vi "ep_Private Inf to Task.vi"(5 "entry values":string[](array[string]), 7 "entry names":string[](array[string]), 8 "error in":errorcluster, 9 "section name":string, 10 "manufacturer name":string, 11 "task in":T1={"file refnums"=[], "Data Object"=refnum, "config info"={"station_name"="", "rec_dev_id"="", "rev_year"=1999.0, "TT"=0, "##A"=0, "##D"=0, "analog channel info"=[], "status channel info"=[], "lf"=-inf, "nrates"=65535, "samp info"=[], "initial timestamp"=timestamp(0 s since 1904-01-01), "trigger timestamp"=timestamp(0 s since 1904-01-01), "ft"=enum."Binary", "timemult"=1.0}, "public inf content"={"Source"="", "Record Type"=enum."Fault", "Phase ID"="", "Event Description"="", "Device ID"="", "Distance of Fault"=-1.0, "Distance Unit"=enum."Miles", "Max_Current"=inf, "Min_Current"=-inf, "Max_Voltage"=inf, "Min_Voltage"=-inf, "EventNoteCount"=0, "Event Information"=[]}, "private inf content"=[], "internal buffers"={"start index"=1, "config to public inf"=enum."disabled", "static config info"="", "static file_des record inf"="", "static file_des channel inf"="", "public inf"="", "private inf"=""}} {"public inf content"."Event Information"."min sample number" max=9999999999; "public inf content"."Event Information"."max sample number" max=9999999999; "config info"."nrates" max=999; "config info"."status channel info"."Dn" min=1 max=999999; "config info"."analog channel info"."An" min=1 max=999999; "config info"."trigger timestamp" format="%<%H:%M:%S%6u\n%d/%m/%Y>T"; "config info"."initial timestamp" format="%<%H:%M:%S%6u\n%d/%m/%Y>T"; "config info"."##D" max=999999; "config info"."##A" max=999999; "config info"."TT" min=1 max=999999; "config info"."rev_year" min=1999.0 max=1999.0}) -> (0 "error out":errorcluster, 3 "task out":T1={"file refnums"=[], "Data Object"=refnum, "config info"={"station_name"="", "rec_dev_id"="", "rev_year"=1999.0, "TT"=0, "##A"=0, "##D"=0, "analog channel info"=[], "status channel info"=[], "lf"=-inf, "nrates"=65535, "samp info"=[], "initial timestamp"=timestamp(0 s since 1904-01-01), "trigger timestamp"=timestamp(0 s since 1904-01-01), "ft"=enum."Binary", "timemult"=1.0}, "public inf content"={"Source"="", "Record Type"=enum."Fault", "Phase ID"="", "Event Description"="", "Device ID"="", "Distance of Fault"=-1.0, "Distance Unit"=enum."Miles", "Max_Current"=inf, "Min_Current"=-inf, "Max_Voltage"=inf, "Min_Voltage"=-inf, "EventNoteCount"=0, "Event Information"=[]}, "private inf content"=[], "internal buffers"={"start index"=1, "config to public inf"=enum."disabled", "static config info"="", "static file_des record inf"="", "static file_des channel inf"="", "public inf"="", "private inf"=""}} {"public inf content"."Event Information"."min sample number" max=9999999999; "public inf content"."Event Information"."max sample number" max=9999999999; "config info"."nrates" max=999; "config info"."status channel info"."Dn" min=1 max=999999; "config info"."analog channel info"."An" min=1 max=999999; "config info"."trigger timestamp" format="%<%H:%M:%S%6u\n%d/%m/%Y>T"; "config info"."initial timestamp" format="%<%H:%M:%S%6u\n%d/%m/%Y>T"; "config info"."##D" max=999999; "config info"."##A" max=999999; "config info"."TT" min=1 max=999999; "config info"."rev_year" min=1999.0 max=1999.0})   [LabVIEW 2011, in "NI_EP_COMTRADE.lvlib"]
uses:
  <vilib>/addons/Electrical Power/File IO/NI_EP_COMTRADE.lvlib
  <vilib>/addons/Electrical Power/File IO/COMTRADE/typedefs/ep_Task.ctl
  <vilib>/addons/Electrical Power/File IO/COMTRADE/typedefs/ep_Config Info.ctl
  <vilib>/addons/Electrical Power/File IO/COMTRADE/typedefs/ep_Analog Channel Info.ctl
  <vilib>/addons/Electrical Power/File IO/COMTRADE/typedefs/ep_Status Channel Info.ctl
  <vilib>/addons/Electrical Power/File IO/COMTRADE/typedefs/ep_File Format.ctl
  <vilib>/addons/Electrical Power/File IO/COMTRADE/typedefs/ep_Public Inf Content.ctl
  <vilib>/addons/Electrical Power/File IO/COMTRADE/typedefs/ep_Public Event Inf.ctl
  <vilib>/addons/Electrical Power/File IO/COMTRADE/typedefs/ep_Private Inf Content.ctl
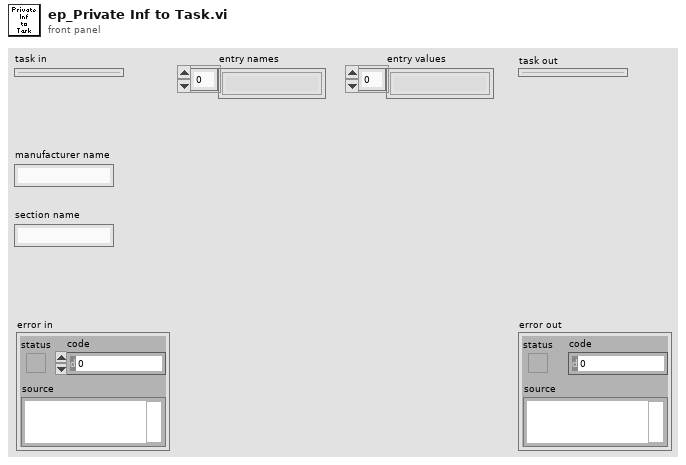
[diagram p1: front panel]
types:
  T1 = typedef "NI_EP_COMTRADE.lvlib/ep_Task.ctl" = cluster{"file refnums":refnum<file>[], "Data Object":refnum<k20>, "config info":T2, "public inf content":T6, "private inf content":T8, "internal buffers":cluster{"start index":u32, "config to public inf":enum16{"disabled", "enabled", "buffered"}, "static config info":string, "static file_des record inf":string, "static file_des channel inf":string, "public inf":string, "private inf":string}}
  T2 = typedef "NI_EP_COMTRADE.lvlib/ep_Config Info.ctl" = cluster{"station_name":string, "rec_dev_id":string, "rev_year":dbl, "TT":u32, "##A":u32, "##D":u32, "analog channel info":T3[], "status channel info":T4[], "lf":sgl, "nrates":u16, "samp info":cluster{"samp":sgl, "endsamp":u32}[], "initial timestamp":timestamp, "trigger timestamp":timestamp, "ft":T5, "timemult":sgl}
  T3 = typedef "NI_EP_COMTRADE.lvlib/ep_Analog Channel Info.ctl" = cluster{"An":u32, "ch_id":string, "ph":string, "ccbm":string, "uu":string, "a":sgl, "b":sgl, "skew":sgl, "min":i32, "max":i32, "primary":sgl, "secondary":sgl, "PS":enum16{"P", "S"}}
  T4 = typedef "NI_EP_COMTRADE.lvlib/ep_Status Channel Info.ctl" = cluster{"Dn":u32, "ch_id":string, "ph":string, "ccbm":string, "Y":bool}
  T5 = typedef "NI_EP_COMTRADE.lvlib/ep_File Format.ctl" = enum16{"ASCII", "Binary"}
  T6 = typedef "NI_EP_COMTRADE.lvlib/ep_Public Inf Content.ctl" = cluster{"Source":string, "Record Type":enum16{"Fault", "Unknown", "Misoperation", "Close", "Trip", "Reclose", "Power swing", "Simulation"}, "Phase ID":string, "Event Description":string, "Device ID":string, "Distance of Fault":dbl, "Distance Unit":enum16{"Miles", "Kilometers", "Percent of line", "Percent of setting", "Ohms"}, "Max_Current":dbl, "Min_Current":dbl, "Max_Voltage":dbl, "Min_Voltage":dbl, "EventNoteCount":u32, "Event Information":T7[]}
  T7 = typedef "NI_EP_COMTRADE.lvlib/ep_Public Event Inf.ctl" = cluster{"channel number":u32, "max value":dbl, "min value":dbl, "max sample number":u64, "min sample number":u64, "max sample text":string[], "min sample text":string[]}
  T8 = typedef "NI_EP_COMTRADE.lvlib/ep_Private Inf Content.ctl" = cluster{"Section Header":string, "Entry Names":string[], "Entry Values":string[]}[]
  T9 = cluster{"Section Header":string, "Entry Names":string[], "Entry Values":string[]}
  T10 = cluster{string, "entry names":string[], "entry values":string[]}
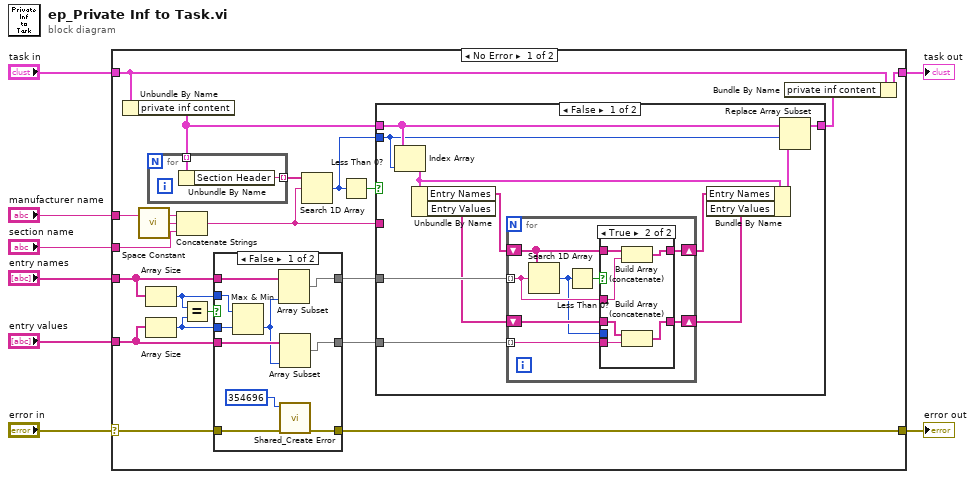
[diagram p0: block diagram]
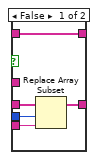
[diagram p3: hidden frame]
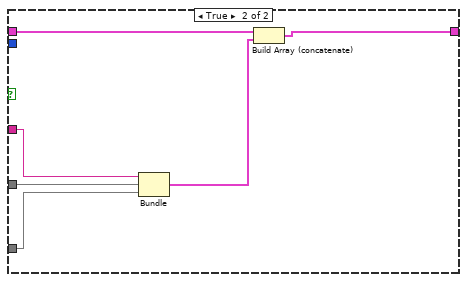
[diagram p4: hidden frame]
diagram:
  n1 = case shown="No Error" "error in" {
    selector: "error in" -> [w10 w80]
    tunnel: "task in" -> [w22 w81]
    tunnel: [w21 w81] -> w6
    tunnel: [w9 w80] -> w1
    tunnel: "manufacturer name" -> [w11 _]
    tunnel: "section name" -> [w12 _]
    tunnel: "entry names" -> [w19 _]
    tunnel: "entry values" -> [w18 _]
    frame No Error {
      n2 = Unbundle By Name(w22) -> ("private inf content"=w25:T8)
      n3 = call <vilib>:"Space Constant.vi"() -> ("String"=w28:string)
      n4 = Array Size(array=w19) -> (size(s)=w17:i32)
      n5 = Array Size(array=w18) -> (size(s)=w16:i32)
      n6 = for {
        tunnel: [w79] -> w27 mode=indexing
        tunnel: w25 -> [w78] mode=indexing
        n7 = Unbundle By Name(w78) -> ("Section Header"=w79:string)
      }
      n8 = Concatenate Strings(w11, w28, w12) -> (w24:string)
      n9 = Equal?(x=w17, y=w16) -> (x = y?=w20:bool)
      n10 = case shown="False" w20 {
        tunnel: [w32 w41] -> w15
        tunnel: w19 -> [w36 w41]
        tunnel: [w33 w40] -> w14
        tunnel: w18 -> [w35 w40]
        tunnel: w17 -> [w38 _]
        tunnel: w16 -> [w37 _]
        tunnel: w10 -> [w30 w39]
        tunnel: [w29 w39] -> w9
        frame False {
          n11 = Max & Min(x=w38, y=w37) -> (min(x,y)=w34:i32)  [unwired: 1 out]
          n12 = Array Subset(array=w36, length=w34) -> (w32:string[])  [unwired: 1 in]
          n13 = Array Subset(array=w35, length=w34) -> (w33:string[])  [unwired: 1 in]
          n14 = call <vilib>:"Shared_Create Error.vi"("error in (no error)"=w30, "error code (0)"=354696 ("code")) -> ("error out"=w29:errorcluster)  [unwired: 9 in]
        }
        frame True {
        }
      }
      n15 = Search 1D Array(1D array=w27, element=w24) -> (index of element=w13:i32)  [unwired: 1 in]
      n16 = Less Than 0?(x=w13) -> (x < 0?=w26:bool)
      n17 = case shown="False" w26 {
        tunnel: w25 -> [w45 w76]
        tunnel: w24 -> [_ w77]
        tunnel: [w44 w75] -> w23
        tunnel: w15 -> [w52 w74]
        tunnel: w14 -> [w50 w73]
        tunnel: w13 -> [w43 _]
        frame False {
          n18 = Index Array(array=w45, index=w43) -> (element=w42:T9)
          n19 = Unbundle By Name(w42) -> ("Entry Names"=w51:string[], "Entry Values"=w49:string[])
          n20 = for {
            tunnel: w52 -> [w57] mode=indexing
            shift-right: [w59] -> w48
            shift-left: w51 -> [w58]
            tunnel: w50 -> [w55] mode=indexing
            shift-right: [w54] -> w47
            shift-left: w49 -> [w56]
            n21 = Search 1D Array(1D array=w58, element=w57) -> (index of element=w53:i32)  [unwired: 1 in]
            n22 = Less Than 0?(x=w53) -> (x < 0?=w60:bool)
            n23 = case shown="True" w60 {
              tunnel: [w61 w71] -> w59
              tunnel: w58 -> [w61 w70]
              tunnel: w57 -> [_ w69]
              tunnel: w56 -> [w64 w68]
              tunnel: w55 -> [w65 w67]
              tunnel: [w63 w66] -> w54
              tunnel: w53 -> [w62 _]
              frame False {
                n24 = Replace Array Subset(array=w64, new element=w65, index=w62) -> (w63:string[])
              }
              frame True {
                n25 = Build Array (concatenate)(w70, w69) -> (w71:string[])
                n26 = Build Array (concatenate)(w68, w67) -> (w66:string[])
              }
            }
          }
          n27 = Bundle By Name(cluster=w42, "Entry Names"=w48, "Entry Values"=w47) -> (w46:T9)
          n28 = Replace Array Subset(array=w45, new element=w46, index=w43) -> (w44:T8)
        }
        frame True {
          n29 = Bundle(w77, "entry names"=w74, "entry values"=w73) -> (w72:T10)  [unwired: 1 in]
          n30 = Build Array (concatenate)(w76, w72) -> (w75:T8)
        }
      }
      n31 = Bundle By Name(cluster=w22, "private inf content"=w23) -> (w21:T1)
    }
    frame Error {
    }
  }
  "task out" <- w6
  "error out" <- w1
